vi "cancel_action.vi"(11 "data":bool) -> ()   [LabVIEW 2024]
uses:
  <vilib>/RTI DDS Toolkit/Types/RTI DDS Advanced Writer Configuration.ctl
  <vilib>/RTI DDS Toolkit/VIs/AdvancedCreateWriter_Bool.vi
  <vilib>/RTI DDS Toolkit/VIs/Write_Bool.vi
  <vilib>/RTI DDS Toolkit/Library/LVDDS_library.lvlib
panel:
  in  "Domain Id":u32
  in  "Topic Name":string="rt/cancel_current_action"
  out "to ROS":bool
  in  "error in (no error)":errorcluster
  in  "Advanced Writer Configuration":T1={"typeName"="std_msgs::msg::dds_::Bool_", "keyName"="", "domainParticipantQoSProfile"="", "dataWriterQoSProfile"="", "forceArrayMapping?"=FALSE, "forceUnboundedString?"=FALSE}
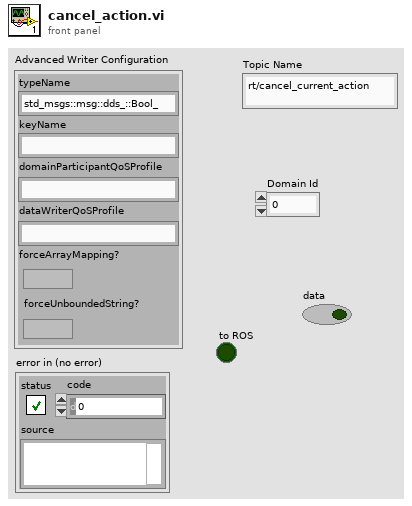
[diagram p1: front panel]
types:
  T1 = typedef "LVDDS_library.lvlib/RTI DDS Advanced Writer Configuration.ctl" = cluster{"typeName":string, "keyName":string, "domainParticipantQoSProfile":string, "dataWriterQoSProfile":string, "forceArrayMapping?":bool, "forceUnboundedString?":bool}
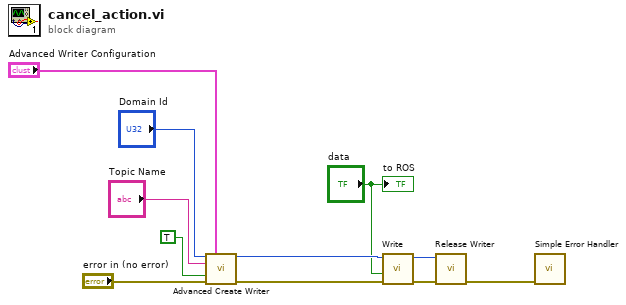
[diagram p0: block diagram]
diagram:
  n1 = call-poly <vilib>:"Advanced Create Writer.vi"("Domain Id"="Domain Id", "Advanced Writer Configuration"="Advanced Writer Configuration", "Topic Name"="Topic Name", "Data Type"=TRUE, "error in (no error)"="error in (no error)") -> ("DDS Object Ref"=w5:u64, "error out"=w4:errorcluster)  [unwired: 9 in]
  n2 = call-poly <vilib>:"Write.vi"("error in (no error)"=w4, "Data"="data", "DDS Object Ref in"=w5) -> ("error out"=w1:errorcluster, "DDS Object Ref out"=w2:u64)  [unwired: 7 in]
  n3 = call <vilib>:"Release Writer.vi"("error in (no error)"=w1, "DDS Object Ref"=w2) -> ("error out"=w11:errorcluster)  [unwired: 9 in]
  n4 = call <vilib>:"Simple Error Handler.vi"("error in (no error)"=w11) -> ()  [unwired: 4 in, 5 out]
  "to ROS" <- "data"
